vi "Preview the image.vi"() -> ()   [LabVIEW 2018]
uses:
  LabViewDVPCamera/LabViewDVPCamera.lvlib
  <vilib>/picture/picture.llb/imagedata.ctl
panel:
  out "Capture frame rate":sgl
  out "Total frame rate":u32
  out "pFrameCount out":T1
  out "frame rate":dbl format="%#.5g"
  out "value":u64
  out "Millisecond timing value 3":u32
  in  "image data":T2 caption="图像数据"
  in  "CloseFlg":i32
  out "handle":u32
  out "new picture":picture caption="新图片"
  in  "CameraList":u16(ring) items=["MGS130M-192.168.0.251"]
  in  "Set":bool
  in  "Close":bool
  in  "Open":bool
  in  "ScanCamera":bool
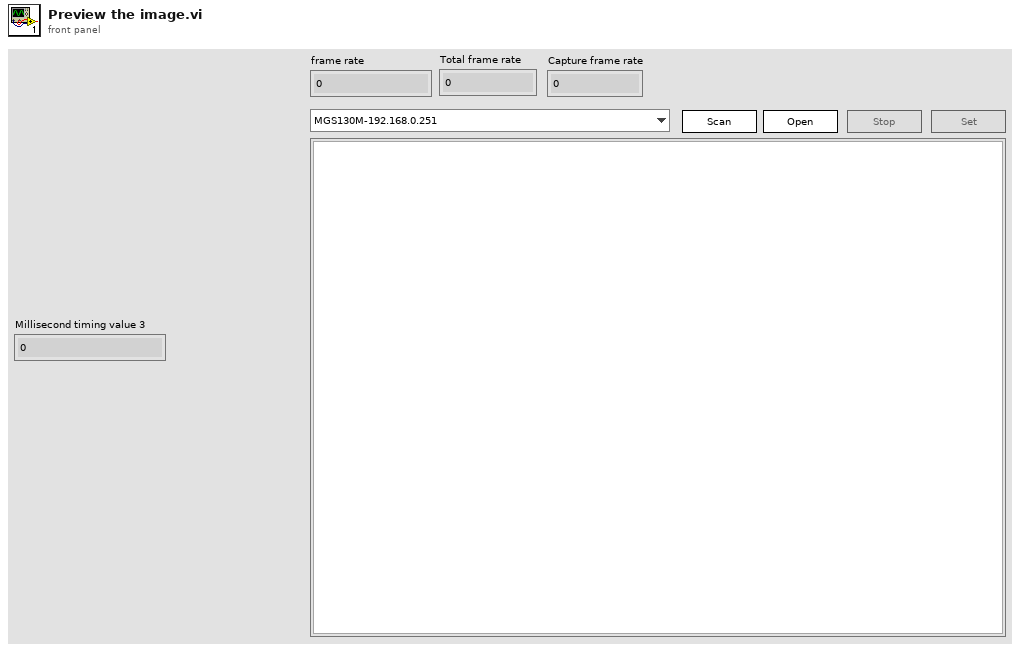
[diagram p1: front panel]
types:
  T1 = cluster{"uFrameCount":u32, "uFrameDrop":u32, "uFrameIgnore":u32, "uFrameError":u32, "uFrameOK":u32, "uFrameOut":u32, "uFrameResend":u32, "uFrameProc":u32, "fFrameRate":sgl, "fProcRate":sgl, "reserved[0]":i32, "reserved[1]":i32, "reserved[2]":i32, "reserved[3]":i32, "reserved[4]":i32, "reserved[5]":i32, "reserved[6]":i32, "reserved[7]":i32, "reserved[8]":i32, "reserved[9]":i32, "reserved[10]":i32, "reserved[11]":i32, "reserved[12]":i32, "reserved[13]":i32, "reserved[14]":i32, "reserved[15]":i32, "reserved[16]":i32, "reserved[17]":i32, "reserved[18]":i32, "reserved[19]":i32, "reserved[20]":i32, "reserved[21]":i32, "reserved[22]":i32, "reserved[23]":i32, "reserved[24]":i32, "reserved[25]":i32, "reserved[26]":i32, "reserved[27]":i32, "reserved[28]":i32, "reserved[29]":i32, "reserved[30]":i32, "reserved[31]":i32}
  T2 = typedef "imagedata.ctl" = cluster{"image type":i32, "image depth":i32, "image":u8[], "mask":u8[], "colors":u32[], "Rectangle":cluster{"left":i16, "top":i16, "right":i16, "bottom":i16}}
  T3 = enum8{"Enabled", "Disabled", "Disabled and Grayed Out"}
  T4 = typedef "LVStringsAndValuesArrayTypeDef_U16.ctl" = cluster{"String":string, "Value":u16}[]
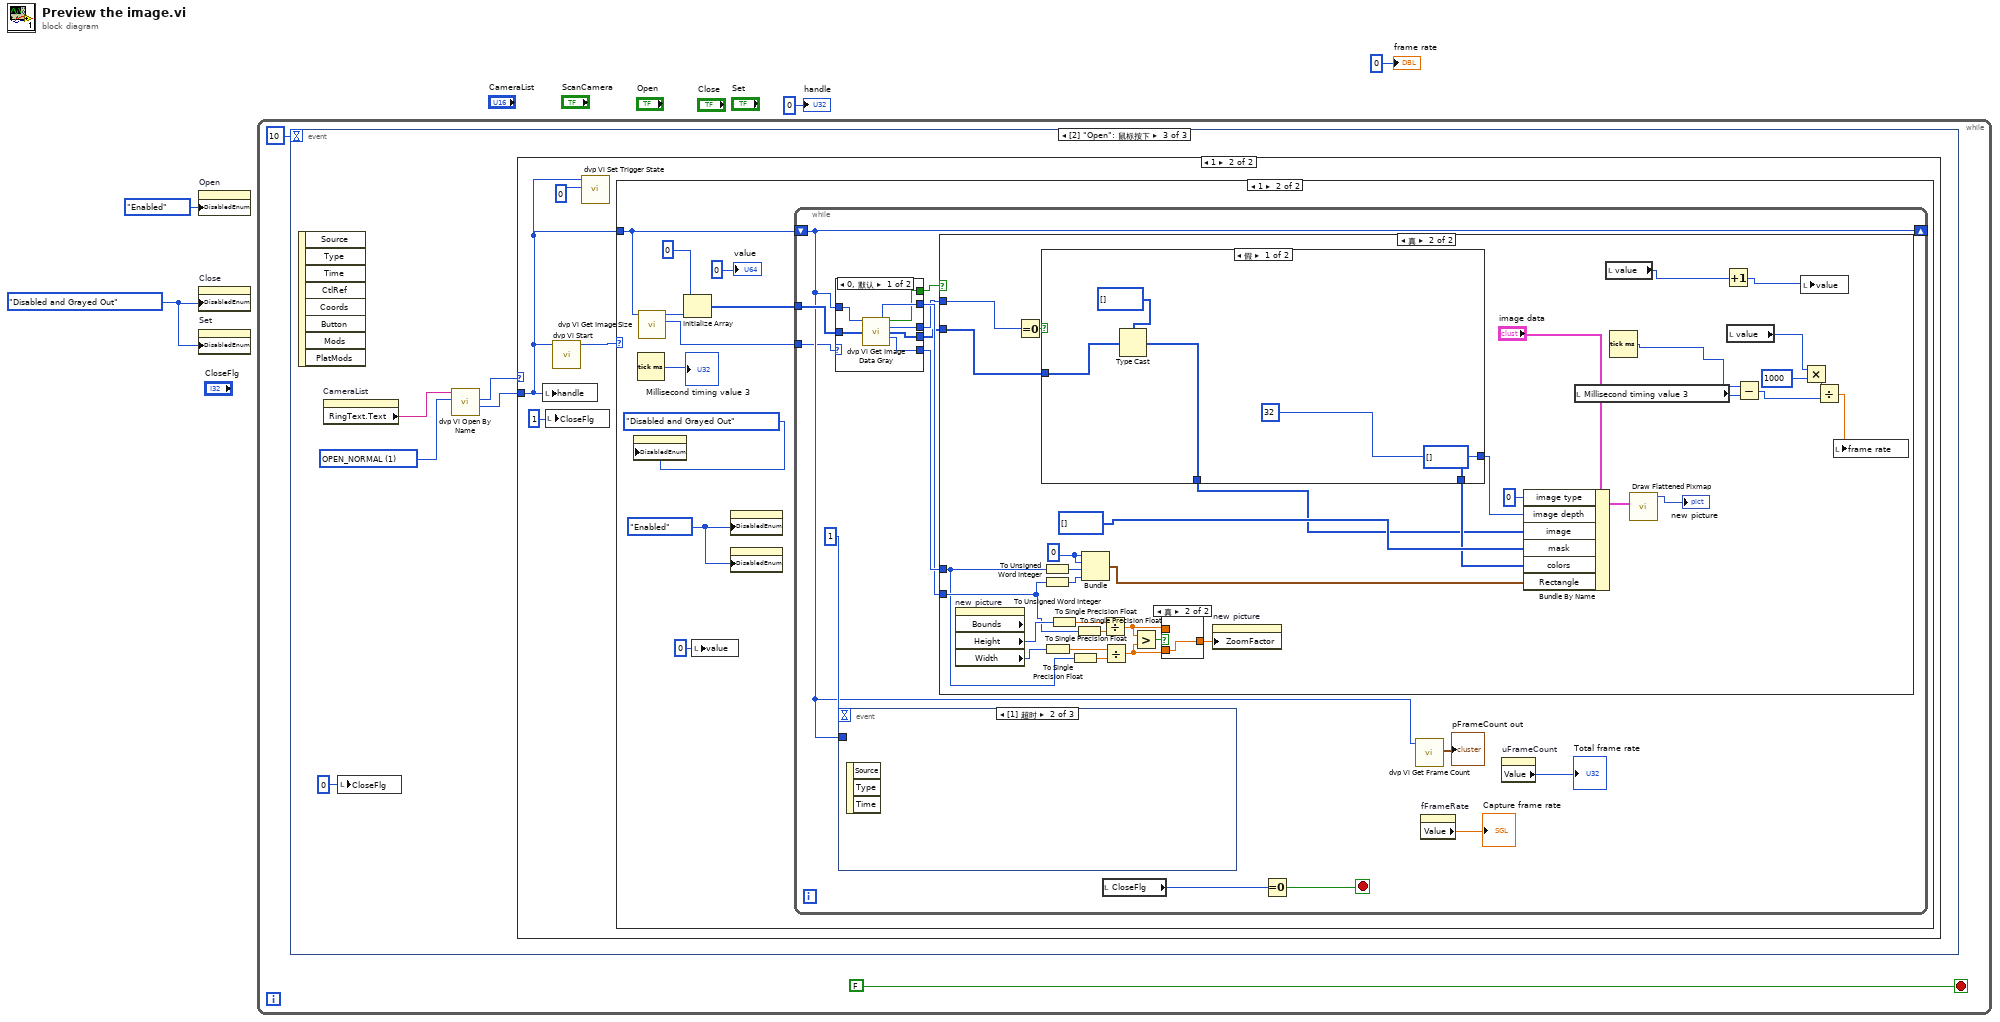
[diagram p0: block diagram]
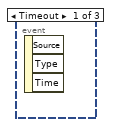
[diagram p2: hidden frame]
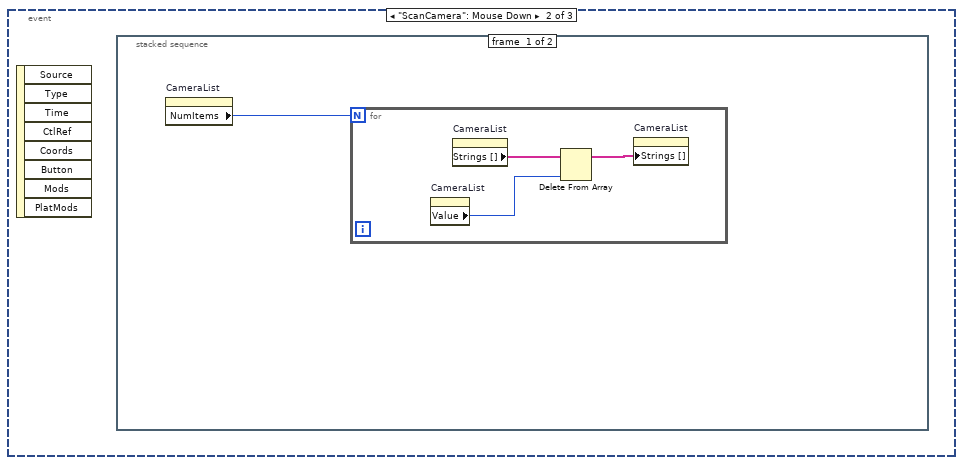
[diagram p3: hidden frame]
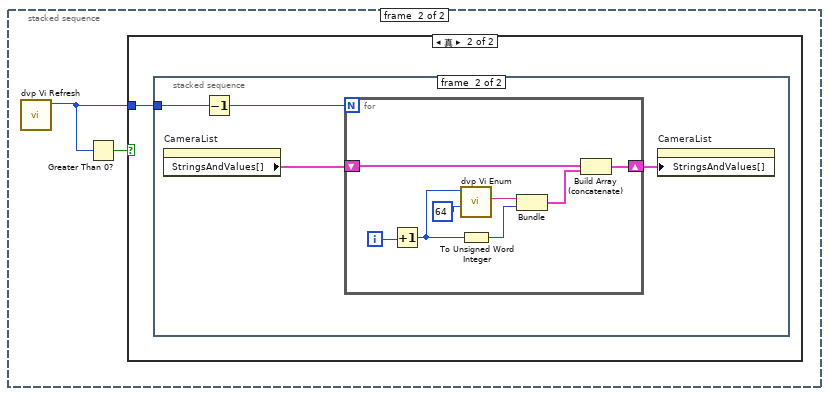
[diagram p4: hidden frame]
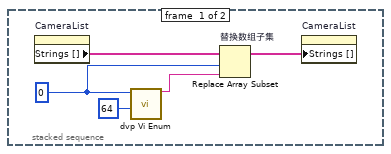
[diagram p6: hidden frame]
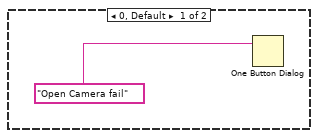
[diagram p7: hidden frame]
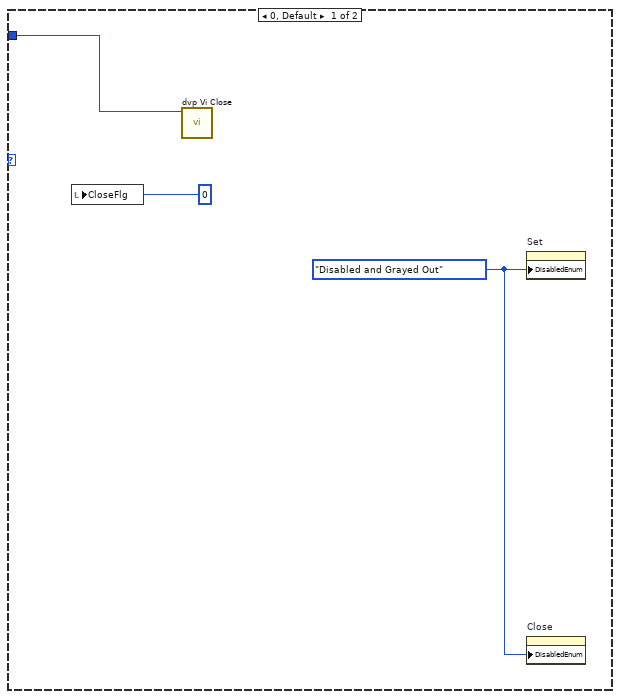
[diagram p8: hidden frame]
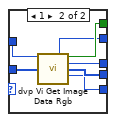
[diagram p9: hidden frame]
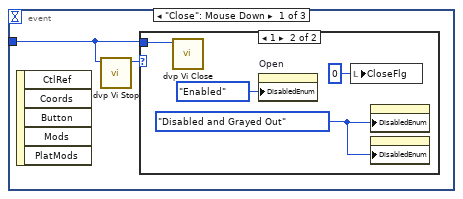
[diagram p10: hidden frame]
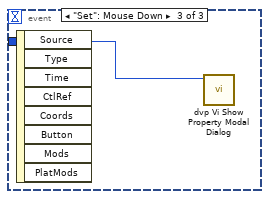
[diagram p12: hidden frame]
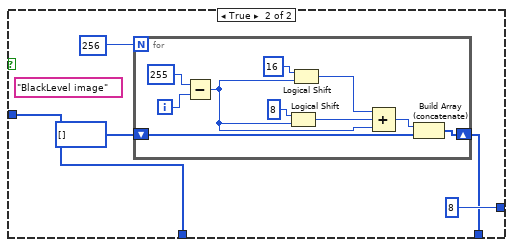
[diagram p15: hidden frame]
diagram:
  w3 = T3."Disabled and Grayed Out" ("禁用")
  n1 = property on="Open" class="Bool"("DisabledEnum"=T3."Enabled" ("禁用")) -> ()  [unwired: 2 in, 2 out]
  n2 = property on="Close" class="Bool"("DisabledEnum"=w3) -> ()  [unwired: 2 in, 2 out]
  n3 = property on="Set" class="Bool"("DisabledEnum"=w3) -> ()  [unwired: 2 in, 2 out]
  n4 = while {
    stop <- FALSE stop-if-true
    n5 = event shown="[2] \"Open\": 鼠标按下" {
      selector: _ -> [_ _ _]
      dyn-events: _ -> [_ _ _]
      timeout: 10 -> [_ _ _]
      event Timeout {
        n6 = event-data() -> ()  [unwired: 1 in, 3 out]
      }
      event "ScanCamera": Mouse Down {
        n7 = event-data() -> ()  [unwired: 1 in, 8 out]
        n8 = stacked-sequence "清除下拉列表的数据" {
          frame #0 {
            n9 = property on="CameraList" class="Ring (严格)"() -> ("NumItems"=w7:u32)  [unwired: 2 in, 2 out]
            n10 = for {
              N: w7 -> [_]
              n11 = property on="CameraList" class="Ring (严格)"() -> ("Value"=w9:u16)  [unwired: 2 in, 2 out]
              n12 = property on="CameraList" class="Ring (严格)"() -> ("Strings []"=w8:string[])  [unwired: 2 in, 2 out]
              n13 = Delete From Array ("删除数组元素")(array=w8, index=w9) -> (array with subset deleted=w10:string[])  [unwired: 1 in, 1 out]
              n14 = property on="CameraList" class="Ring (严格)"("Strings []"=w10) -> ()  [unwired: 2 in, 2 out]
            }
          }
          frame #1 {
            n15 = call "dvp Vi Refresh.vi"() -> ("pCount out"=w12:u32)  [unwired: 10 in, 1 out]
            n16 = Greater Than 0?(x=w12) -> (x > 0?=w11:bool)
            n17 = case shown="真" w11 {
              tunnel: w12 -> [_ w13]
              frame False {
              }
              frame True {
                n18 = stacked-sequence {
                  tunnel: w13 -> [_ w20]
                  frame #0 {
                    w14 = u32 0 ("index")
                    n19 = property on="CameraList" class="Ring (严格)"() -> ("Strings []"=w17:string[])  [unwired: 2 in, 2 out]
                    n20 = call "dvp Vi Enum.vi"("unSize"=u32 64, "index"=w14) -> ("friendlyName out"=w16:string)  [unwired: 8 in, 1 out]
                    n21 = Replace Array Subset "替换数组子集"(array=w17, new element=w16, index=w14) -> (w18:string[])
                    n22 = property on="CameraList" class="Ring (严格)"("Strings []"=w18) -> ()  [unwired: 2 in, 2 out]
                  }
                  frame #1 {
                    n23 = property on="CameraList" class="Ring (严格)"() -> ("StringsAndValues[]"=w22:T4)  [unwired: 2 in, 2 out]
                    n24 = Decrement(x=w20) -> (x-1=w19:u32)
                    n25 = for {
                      N: w19 -> [_]
                      shift-right: [w29] -> w21
                      shift-left: w22 -> [w27]
                      i -> [w24]
                      n26 = Increment(x=w24) -> (x+1=w23:i32)
                      n27 = call "dvp Vi Enum.vi"("unSize"=u32 64, "index"=w23) -> ("friendlyName out"=w30:string)  [unwired: 8 in, 1 out]
                      n28 = To Unsigned Word Integer(number=w23) -> (unsigned 16bit integer=w26:u16)
                      n29 = Bundle("friendlyName out"=w30, w26) -> (w28:cluster{"friendlyName out":string, u16})  [unwired: 1 in]
                      n30 = Build Array (concatenate)(w27, w28) -> (w29:T4)
                    }
                    n31 = property on="CameraList" class="Ring (严格)"("StringsAndValues[]"=w21) -> ()  [unwired: 2 in, 2 out]
                  }
                }
              }
            }
          }
        }
      }
      event "Open": Mouse Down {
        w33 = u32 1 items=["OPEN_OFFLINE", "OPEN_NORMAL"] ("type")
        n32 = event-data() -> ()  [unwired: 1 in, 8 out]
        n33 = property on="CameraList" class="Ring (严格)"() -> ("RingText.Text"=w32:string)  [unwired: 2 in, 2 out]
        n34 = local write "CloseFlg"(0 ("CloseFlg")) -> ()
        n35 = call "dvp Vi Open By Name.vi"("type"=w33, "friendlyName"=w32) -> ("pHandle out"=w35:u32, "function return"=w34:u32)  [unwired: 7 in, 1 out]
        n36 = case shown="1" w34 {
          tunnel: w35 -> [_ w37]
          frame 0, Default {
            n37 = One Button Dialog(message="Open Camera fail" ("消息")) -> ()  [unwired: 1 in, 1 out]
          }
          frame 1 {
            n38 = local write "handle"(w37) -> ()
            n39 = local write "CloseFlg"(1 ("CloseFlg")) -> ()
            n40 = call "dvp Vi Start.vi"("handle"=w37) -> ("function return"=w39:u32)  [unwired: 10 in]
            n41 = call "dvp Vi Set Trigger State.vi"("TriggerState"=0, "handle"=w37) -> ()  [unwired: 9 in, 1 out]
            n42 = case shown="1" w39 {
              tunnel: w37 -> [w43 w49]
              frame 0, Default {
                w42 = T3."Disabled and Grayed Out" ("禁用")
                n43 = local write "CloseFlg"(0 ("CloseFlg")) -> ()
                n44 = call "dvp Vi Close.vi"("handle"=w43) -> ()  [unwired: 10 in, 1 out]
                n45 = property on="Set" class="Bool"("DisabledEnum"=w42) -> ()  [unwired: 2 in, 2 out]
                n46 = property on="Close" class="Bool"("DisabledEnum"=w42) -> ()  [unwired: 2 in, 2 out]
              }
              frame 1 {
                w53 = T3."Enabled" ("禁用")
                n47 = property on="Open" class="Bool"("DisabledEnum"=T3."Disabled and Grayed Out" ("禁用")) -> ()  [unwired: 2 in, 2 out]
                n48 = Tick Count (ms)() -> (millisecond timer value=→"Millisecond timing value 3":u32)
                n49 = call "dvp Vi Get Image Size.vi"("handle"=w49) -> ("pformat out"=w45:i32, "function return"=w48:u32)  [unwired: 9 in]
                n50 = Initialize Array(u32 0 ("元素"), w48) -> (w50:u32[])
                n51 = local write "value"(u64 0 ("数值")) -> ()
                n52 = property on="Set" class="Bool"("DisabledEnum"=w53) -> ()  [unwired: 2 in, 2 out]
                n53 = property on="Close" class="Bool"("DisabledEnum"=w53) -> ()  [unwired: 2 in, 2 out]
                n54 = while {
                  shift-right: [w60] -> _
                  shift-left: w49 -> [w60]
                  tunnel: w50 -> [w61]
                  tunnel: w45 -> [w59]
                  stop <- w66 stop-if-true
                  n55 = case shown="0, 默认" w59 {
                    tunnel: w61 -> [w74 w81]
                    tunnel: w60 -> [w73 w80]
                    tunnel: [w69 w79] -> w55
                    tunnel: [w71 w78] -> w54
                    tunnel: [w70 w77] -> w56
                    tunnel: [w72 w76] -> w57
                    tunnel: [w68 w75] -> w58
                    frame 0, Default {
                      n56 = call "dvp Vi Get Image Data Gray.vi"("handle"=w73, "pbuffer"=w74) -> ("piHeight out"=w72:i32, "function return"=w69:bool, "pformat out"=w70:i32, "pbuffer out"=w71:u8[], "piWidth out"=w68:i32)  [unwired: 9 in]
                    }
                    frame 1 {
                      n57 = call "dvp Vi Get Image Data Rgb.vi"("handle"=w80, "pbuffer"=w81) -> ("piHeight out"=w76:i32, "function return"=w79:bool, "pformat out"=w77:i32, "pbuffer out"=w78:u32[], "piWidth out"=w75:i32)  [unwired: 9 in]
                    }
                  }
                  n58 = event shown="[1] 超时" {
                    selector: _ -> [_ _ _]
                    dyn-events: _ -> [_ _ _]
                    timeout: 1 -> [_ _ _]
                    tunnel: w60 -> [w82 _ w88]
                    event "Close": Mouse Down {
                      n59 = event-data() -> ()  [unwired: 1 in, 5 out]
                      n60 = call "dvp Vi Stop.vi"("handle"=w82) -> ("function return"=w83:u32)  [unwired: 10 in]
                      n61 = case shown="1" w83 {
                        tunnel: w82 -> [_ w85]
                        frame 0, Default {
                        }
                        frame 1 {
                          w84 = T3."Disabled and Grayed Out" ("禁用")
                          n62 = call "dvp Vi Close.vi"("handle"=w85) -> ()  [unwired: 10 in, 1 out]
                          n63 = property on="Open" class="Bool"("DisabledEnum"=T3."Enabled" ("禁用")) -> ()  [unwired: 2 in, 2 out]
                          n64 = local write "CloseFlg"(0 ("CloseFlg")) -> ()
                          n65 = property on="Close" class="Bool"("DisabledEnum"=w84) -> ()  [unwired: 2 in, 2 out]
                          n66 = property on="Set" class="Bool"("DisabledEnum"=w84) -> ()  [unwired: 2 in, 2 out]
                        }
                      }
                    }
                    event Timeout {
                      n67 = event-data() -> ()  [unwired: 1 in, 3 out]
                    }
                    event "Set": Mouse Down {
                      n68 = event-data() -> ()  [unwired: 1 in, 8 out]
                      n69 = call "dvp Vi Show Property Modal Dialog.vi"("handle"=w88) -> ()  [unwired: 10 in, 1 out]
                    }
                  }
                  n70 = case shown="真" w55 {
                    tunnel: w54 -> [_ w91]
                    tunnel: w58 -> [_ w92]
                    tunnel: w57 -> [_ w93]
                    tunnel: w56 -> [_ w121]
                    frame False {
                    }
                    frame True {
                      w124 = u16 0
                      n71 = property on="new picture" class="Pict" props=["Bounds", "Height", "Width"]() -> ("Height"=w94:u32, "Width"=w95:u32)  [unwired: 2 in, 3 out]
                      n72 = Equal To 0?(x=w121) -> (x = 0?=w120:bool)
                      n73 = case shown="假" w120 {
                        tunnel: [32 u8 8 ("image depth")] -> w117
                        tunnel: [i32[] [] ("数组") w133] -> w115
                        tunnel: w91 -> [w128 w132]
                        tunnel: [w127 w132] -> w90
                        frame False {
                          n74 = Type Cast(type=u8[] [], x=w128) -> (*(type *) &x=w127:u8[])
                        }
                        frame True {
                          (unwired) "BlackLevel image"
                          n75 = for {
                            N: 256 -> [_]
                            shift-right: [w141] -> w133
                            shift-left: i32[] [] ("数组") -> [w140]
                            i -> [w137]
                            n76 = Subtract(x=255, y=w137) -> (x-y=w138:i32)
                            n77 = Logical Shift(y=i16 8, x=w138) -> (x << y=w143:i32)
                            n78 = Logical Shift(y=16 ("x"), x=w138) -> (x << y=w144:i32)
                            n79 = Compound Arithmetic op=ADD(w144, w143, w138) -> (w142:i32)
                            n80 = Build Array (concatenate)(w142, w140) -> (w141:i32[])
                          }
                        }
                      }
                      n81 = To Unsigned Word Integer(number=w92) -> (unsigned 16bit integer=w123:u16)
                      n82 = To Unsigned Word Integer(number=w93) -> (unsigned 16bit integer=w122:u16)
                      n83 = To Single Precision Float(number=w95) -> (single precision float=w102:sgl)
                      n84 = To Single Precision Float(number=w94) -> (single precision float=w96:sgl)
                      n85 = To Single Precision Float(number=w92) -> (single precision float=w98:sgl)
                      n86 = To Single Precision Float(number=w93) -> (single precision float=w97:sgl)
                      n87 = Bundle ("图像尺寸")(w124, w124, w123, w122) -> (w114:cluster{u16, u16, u16, u16})  [unwired: 1 in]
                      n88 = Divide(x=w96, y=w97) -> (x/y=w100:sgl)
                      n89 = Divide(x=w102, y=w98) -> (x/y=w101:sgl)
                      n90 = Greater?(x=w100, y=w101) -> (0:w99:bool)
                      n91 = case shown="真" w99 {
                        tunnel: w100 -> [w125 _]
                        tunnel: w101 -> [_ w126]
                        tunnel: [w125 w126] -> w103
                        frame False {
                        }
                        frame True {
                        }
                      }
                      n92 = property on="new picture" class="Pict"("ZoomFactor"=w103) -> ()  [unwired: 2 in, 2 out]
                      n93 = Bundle By Name(cluster="image data", "image type"=0, "image depth"=w117, "image"=w90, "mask"=u8[] [] ("无符号8位数组"), "colors"=w115, "Rectangle"=w114) -> (w118:T2)
                      n94 = local read "Millisecond timing value 3"() -> (w106:u32)
                      n95 = local read "value"() -> (w109:u64)
                      n96 = Tick Count (ms)() -> (millisecond timer value=w107:u32)
                      n97 = call <vilib>:"Draw Flattened Pixmap.vi"("image data"=w118) -> ("new picture"=→"new picture":picture)  [unwired: 8 in]
                      n98 = Increment(x=w109) -> (x+1=w108:u64)
                      n99 = local read "value"() -> (w105:u64)
                      n100 = Subtract(x=w107, y=w106) -> (x-y=w112:u32)
                      n101 = local write "value"(w108) -> ()
                      n102 = Multiply(x=w105, y=u64 1000) -> (x*y=w110:u64)
                      n103 = Divide(x=w110, y=w112) -> (x/y=w104:dbl)
                      n104 = local write "frame rate"(w104) -> ()
                    }
                  }
                  n105 = local read "CloseFlg"() -> (w65:i32)
                  n106 = Equal To 0?(x=w65) -> (x = 0?=w66:bool)
                  n107 = call "dvp Vi Get Frame Count.vi"("handle"=w60) -> ("pFrameCount out"=→"pFrameCount out":T1)  [unwired: 9 in, 1 out]
                  n108 = property on="fFrameRate" class="DigNum (严格)"() -> ("Value"=→"Capture frame rate":sgl)  [unwired: 2 in, 2 out]
                  n109 = property on="uFrameCount" class="DigNum (严格)"() -> ("Value"=→"Total frame rate":u32)  [unwired: 2 in, 2 out]
                }
                "value" <- u64 0
              }
            }
          }
        }
      }
    }
  }
  "handle" <- u32 0 ("handle")
  "frame rate" <- 0
